vi "Read_Balance.vi"() -> (0 "string":string, 1 "Stable?":bool, 2 "Mass (dbl)":dbl, 3 "No Error?":bool, 4 "Error?":bool)   [LabVIEW 2019]
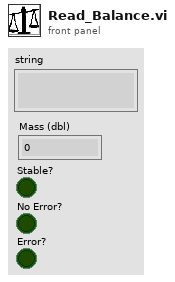
[diagram p1: front panel]
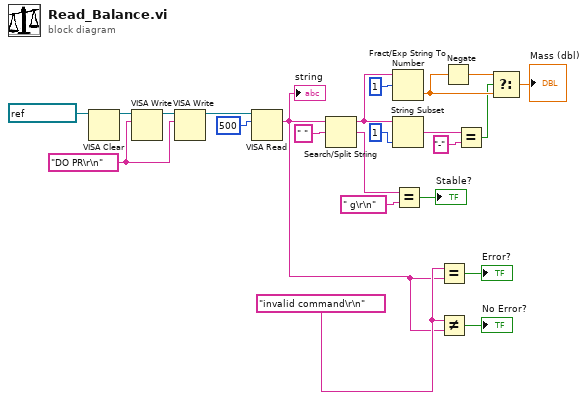
[diagram p0: block diagram]
diagram:
  w4 = "invalid command\r\n"
  w12 = "DO PR\r\n" ("write buffer")
  n1 = VISA Clear(VISA resource name=refnum<visa-resource-name> "COM11") -> (VISA resource name out=w10:refnum<visa-resource-name>)  [unwired: 1 in, 1 out]
  n2 = VISA Write(VISA resource name=w10, write buffer=w12) -> (VISA resource name out=w14:refnum<visa-resource-name>)  [unwired: 1 in, 2 out]
  n3 = VISA Write(VISA resource name=w14, write buffer=w12) -> (VISA resource name out=w13:refnum<visa-resource-name>)  [unwired: 1 in, 2 out]
  n4 = VISA Read(VISA resource name=w13, byte count=u32 500) -> (read buffer=w3:string)  [unwired: 1 in, 3 out]
  "string" <- w3
  n5 = Search/Split String(string=w3, search string/char (-)=" ") -> (substring before match=w9:string, match + rest of string=w7:string)  [unwired: 1 in, 1 out]
  n6 = Fract/Exp String To Number(string=w9, offset=1) -> (number=w20:dbl)  [unwired: 2 in, 1 out]
  n7 = String Subset(string=w9, length (rest)=1 ("length (rest)")) -> (substring=w18:string)  [unwired: 1 in]
  n8 = Equal?(x=w7, y=" g\r\n") -> (x = y?=→"Stable?":bool)
  n9 = Equal?(x=w4, y=w3) -> (x = y?=→"Error?":bool)
  n10 = Not Equal?(x=w4, y=w3) -> (x != y?=→"No Error?":bool)
  n11 = Negate(x=w20) -> (-x=w21:dbl)
  n12 = Equal?(x=w18, y="-") -> (x = y?=w16:bool)
  n13 = Select(t=w21, s=w16, f=w20) -> (s? t:f=→"Mass (dbl)":dbl)
